vi "Channel type to name.vi"(8 "Error In":errorcluster, 11 "Channel type":T1=enum."Flow meter") -> (0 "Error Out":errorcluster, 3 "Name":string)   [LabVIEW 2015]
uses:
  Channel type.ctl
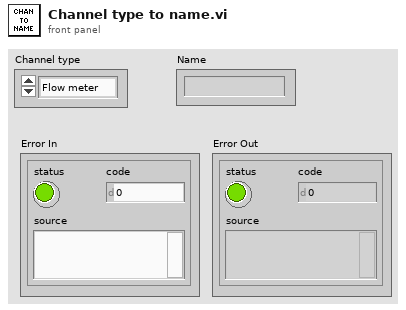
[diagram p1: front panel]
types:
  T1 = typedef "Channel type.ctl" = enum16{"Volts", "Flow meter", "Tank pressure", "Dewar level", "Raw ADC"}
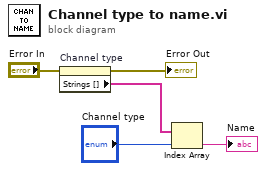
[diagram p0: block diagram]
diagram:
  n1 = property on="Channel type" class="Enum (strict)"(error in="Error In") -> (error out=→"Error Out":errorcluster, "Strings []"=w3:string[])  [unwired: 1 in, 1 out]
  n2 = Index Array(array=w3, index="Channel type") -> (element=→"Name":string)
